vi "Send String Message.vi"(8 "error in (no error)":errorcluster, 10 "Data To Write":string, 11 "SessionHandler in":refnum<class "SessionHandler.lvclass">) -> (0 "error out":errorcluster, 3 "SessionHandler out":refnum<class "SessionHandler.lvclass">)   [LabVIEW 2019, in "Network Sink.lvlib" / "SessionHandler.lvclass"]
uses:
  <vilib>/gpm_packages/@cs/event-logger/Source/Network Sink/SessionHandler/SessionHandler.lvclass
  <vilib>/gpm_packages/@cs/event-logger/Source/Network Sink/SessionHandler/SessionHandler.lvclass/SessionHandler.ctl
  <vilib>/gpm_packages/@cs/Network-Sink/Source/Network Interface/Network Interface/Network Interface.lvclass/Network Interface.ctl
  <vilib>/gpm_packages/@cs/Network-Sink/Source/Network Interface/Message Queue/Message Queue.lvclass/Message Queue.ctl
  <vilib>/gpm_packages/@cs/Network-Sink/Source/Network Interface/Network Interface/Write.vi/dc351019-4f29-47b2-a483-8ae26d0321a6.vi
  <vilib>/gpm_packages/@cs/Network-Sink/Source/Network Interface/Message Queue/Protected Enqueue.vi
  <vilib>/gpm_packages/@cs/Network-Sink/Source/Network Interface/Network Interface/Network Interface.lvclass
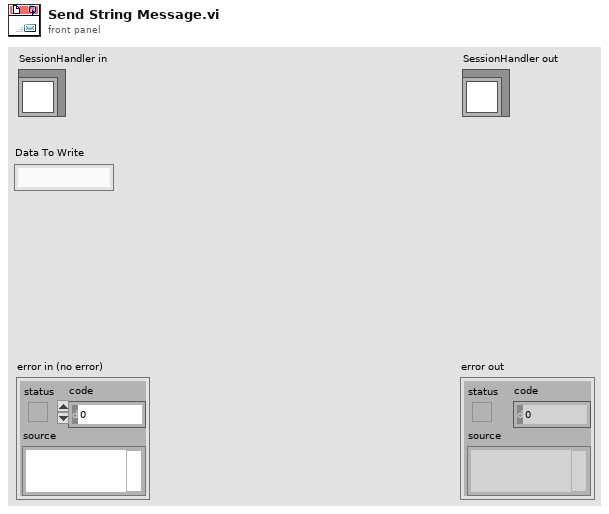
[diagram p1: front panel]
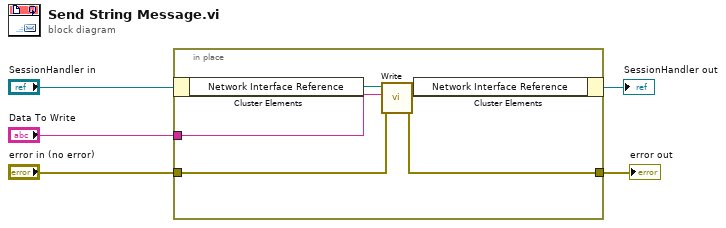
[diagram p0: block diagram]
diagram:
  n1 = in-place {
    in-place-border: "error in (no error)" -> [w10]
    in-place-border: [w9] -> w4
    in-place-border: "Data To Write" -> [w8]
    n2 = in-place-cluster #1("SessionHandler in") -> ("Network Interface Reference"=w7:refnum<data-value>)
    n3 = call <vilib>:"Write.vi"("error in (no error)"=w10, "Data To Write"=w8, "Network Interface"=w7) -> ("error out"=w9:errorcluster, "Network Interface Out"=w6:refnum<data-value>)  [unwired: 7 in]
    n4 = in-place-cluster #1("Network Interface Reference"=w6) -> (→"SessionHandler out":refnum<class "SessionHandler.lvclass">)
  }
  "error out" <- w4
